vi "S8300E_Chk_TEMPERATURE_WIH.vi"() -> ()   [LabVIEW 2011]
uses:
  Instance          16 28Saved   KT300WR2_TP125B_PCBA .vi
  Instance          20 28Saved   KT300WR2_TP125B_PCBA .vi
panel:
  out "history_log":string
  out "VISA resource name out":refnum<visa-resource-name>
  out "SEARCHING Test Item":string[](array[string])
  out "SFCS_Network Ok?":bool=TRUE
  out "log_measured Voltage":string
  out "begin time":u32
  out "All Pass?":bool=TRUE
  out "Result(測試總結果)":bool
  out "Total TP":i32
  out "record(s)":T1(array[cluster])
  out "狀況":string
  out "Test Result (測試結果)":T2(array[cluster])
  # "S8300E 溫度Test Points Check"
  # "2015-6-1"
  # "Error Code\nCPU1\nCPU2\nPCH\nDDR3-1T\nDDR3-2T\nMB"
types:
  T1 = cluster{"TestPoint_Name":string, "Lower Limit Voltage":dbl, "High Limit Voltage":dbl, cluster{"Relay3 Name":string, "Relay3H/L":bool}[], "Measure Ai name":string}[]
  T2 = cluster{"Test Item":string, "SPEC MIN C":dbl, "SPEC MAX C":dbl, "Measured C":dbl, bool}[]
  T3 = enum16{"open", "replace", "create", "open or create", "replace or create", "replace or create with confirmation"}
  T4 = cluster{"Test Item":string, "SPEC MIN V":dbl, "SPEC MAX V":dbl, "Measured V":dbl, bool}[]
  T5 = cluster{"Test Item":string, "SPEC MIN C":dbl, "SPEC MAX C":dbl, "Measured C":dbl, bool}
  T6 = cluster{"TestPoint_Name":string, "Lower Limit Voltage":dbl, "High Limit Voltage":dbl, cluster{"Relay3 Name":string, "Relay3H/L":bool}[], "Measure Ai name":string}
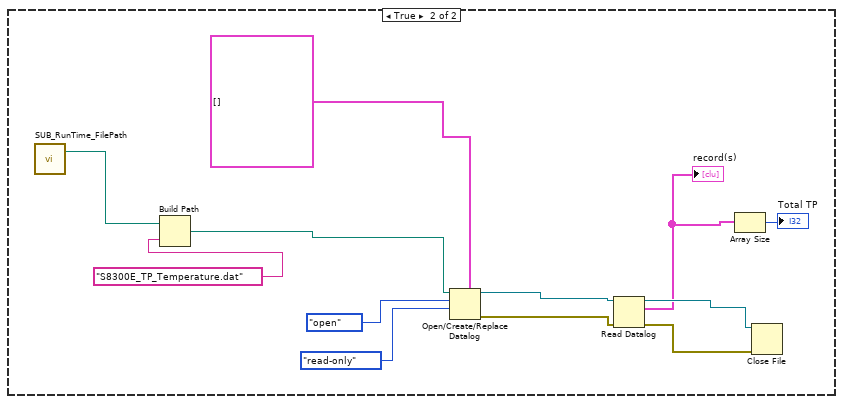
[diagram p2: hidden frame]
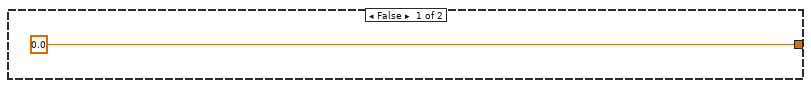
[diagram p6: hidden frame]
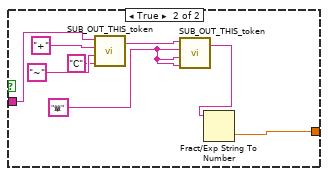
[diagram p7: hidden frame]
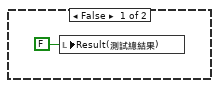
[diagram p9: hidden frame]
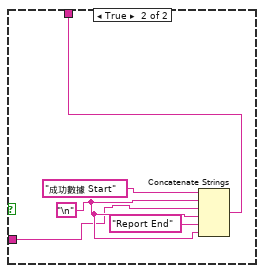
[diagram p10: hidden frame]
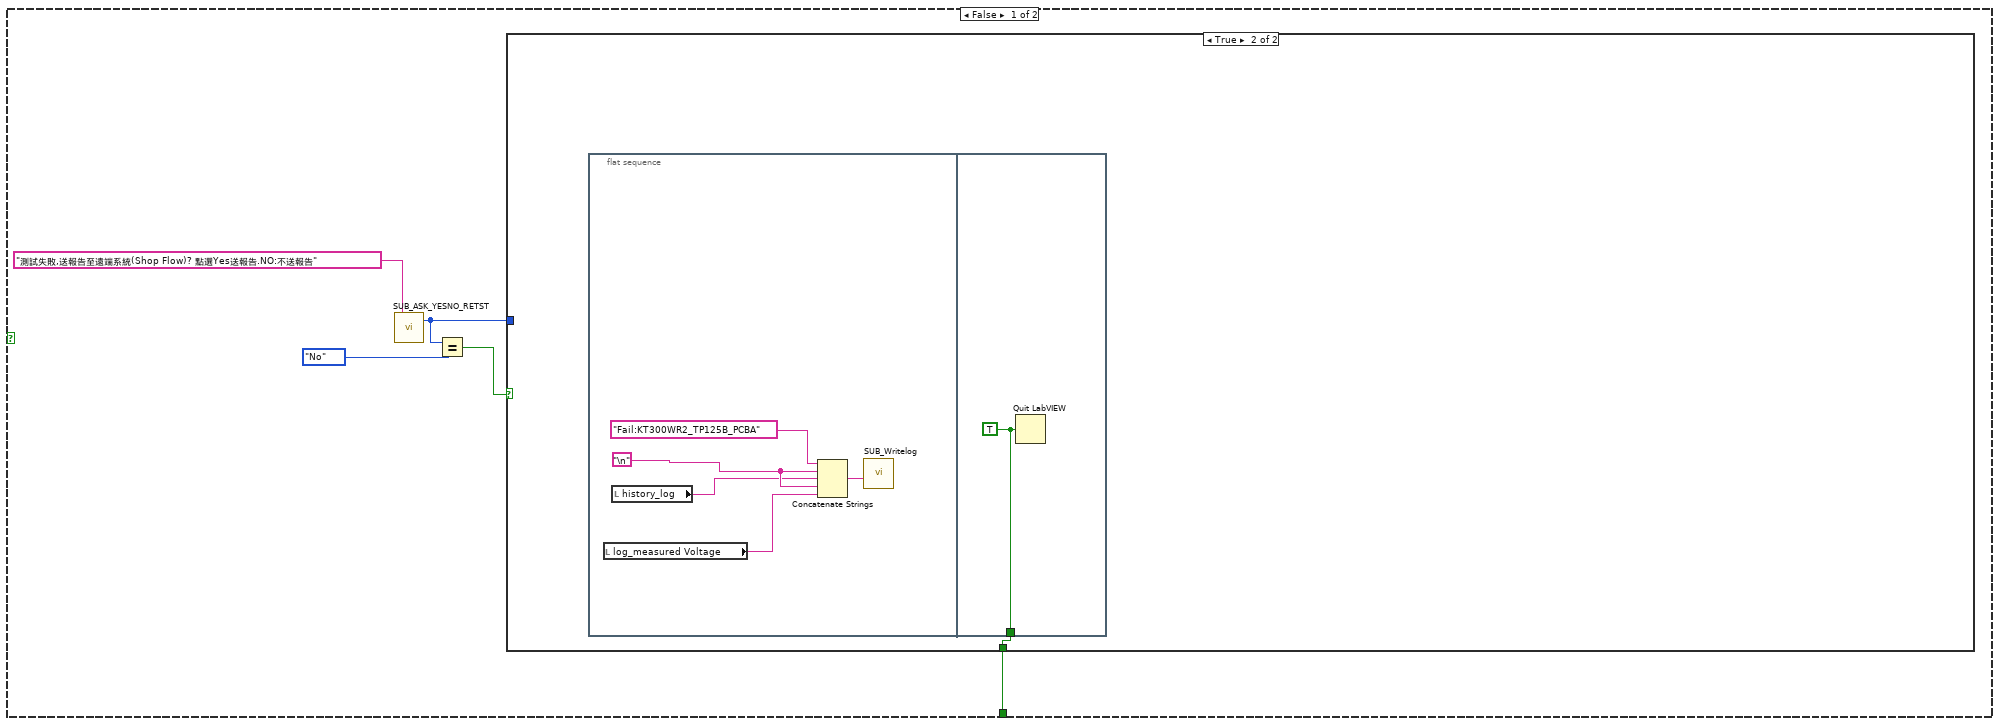
[diagram p11: hidden frame]
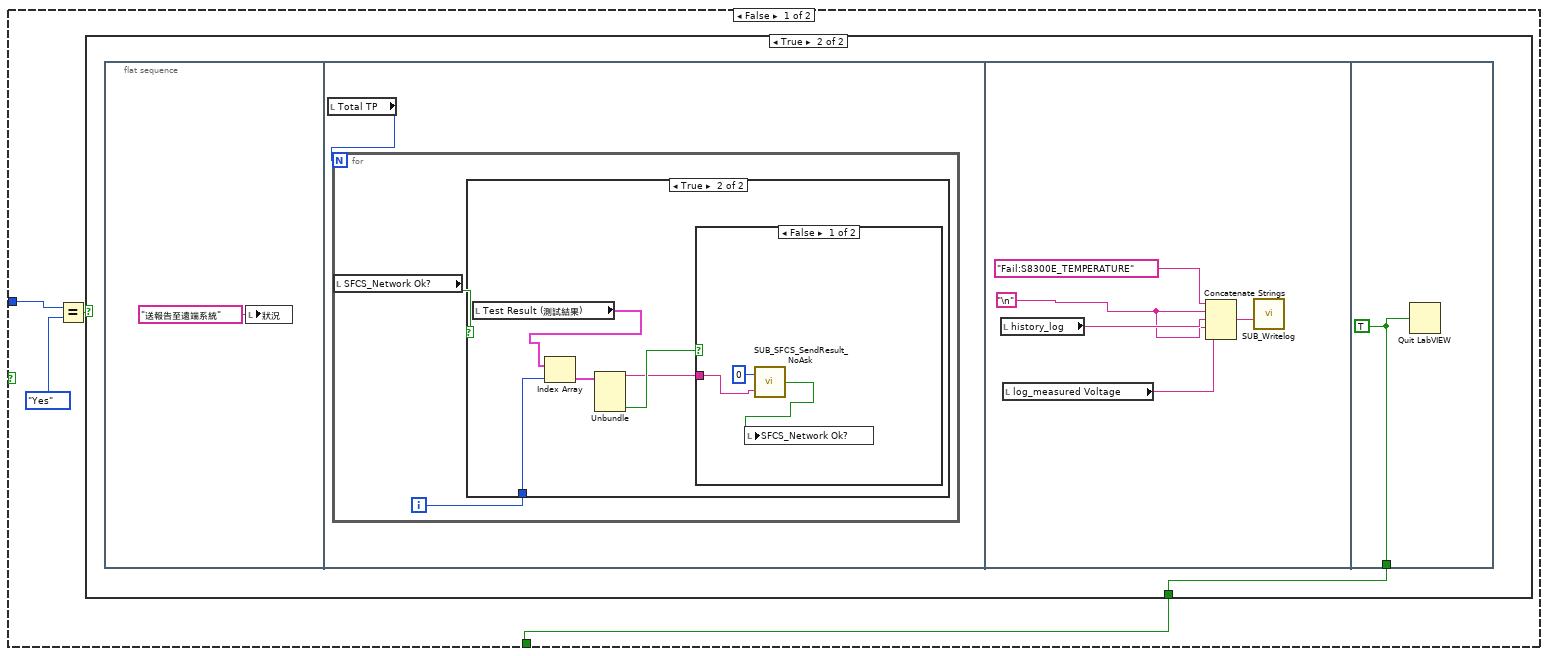
[diagram p12: hidden frame]
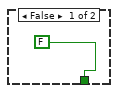
[diagram p13: hidden frame]
diagram:
  n1 = while {
    shift-right: [w4] -> _
    shift-left: "" -> [w3]
    stop <- w6 stop-if-true
    n2 = flat-sequence {
      tunnel: [w48] -> w5
      tunnel: w5 -> [w75]
      tunnel: [w167] -> w2
      tunnel: [w182] -> w6
      frame #0 {
        n3 = Tick Count (ms)() -> (millisecond timer value=→"begin time":u32)
      }
      frame #1 {
        n4 = property on="Result(測試總結果)" class="Bool (strict)"("Visible"=FALSE) -> ()  [unwired: 2 in, 2 out]
        n5 = property on="狀況" class="Str"("Blinking"=TRUE) -> ()  [unwired: 2 in, 2 out]
        "SFCS_Network Ok?" <- TRUE
        "狀況" <- ""
        "Result(測試總結果)" <- FALSE ("Result(測試總結果)")
        "All Pass?" <- TRUE
      }
      frame #2 {
        n6 = call "SUB_SearchFile_inFolder.vi"("Search Filename in Folder"="S8300E_TP_Temperature.dat" ("name or relative path")) -> ("File Existing True/Flase"=w14:bool)  [unwired: 1 in]
        n7 = case shown="False" w14 {
          frame False {
            n8 = flat-sequence {
              frame #0 {
                n9 = call "Display Message to User"() -> ()  [unwired: 10 in, 2 out]
              }
              frame #1 {
                n10 = call "SUB_Writelog.vi"("Pass/Fail"="Fail:S8300E_Chk_TEMPERATURE") -> ()  [unwired: 2 in]
              }
              frame #2 {
                n11 = Quit LabVIEW(quit? (T)=TRUE) -> ()
              }
            }
          }
          frame True {
            n12 = call "SUB_RunTime_FilePath.vi"() -> ("stripped path"=w19:path)  [unwired: 3 in]
            n13 = Build Path(base path=w19, name or relative path="S8300E_TP_Temperature.dat") -> (appended path=w26:path)
            n14 = Open/Create/Replace Datalog(5:T1 [] ("DatalogType"), 9:enum16{"read/write", "read-only", "write-only"}."read-only" ("access (0:read/write)"), 10:T3."open" ("operation (0:open)"), 11:w26) -> (0:w23:errorcluster, 3:w22:refnum<k1>)  [unwired: 2 in, 1 out]
            n15 = Read Datalog(4:w23, 7:w22) -> (0:w25:errorcluster, 2:w21:T1, 3:w24:refnum<k1>)  [unwired: 1 in]
            "record(s)" <- w21
            n16 = Array Size(array=w21) -> (size(s)=→"Total TP":i32)
            n17 = Close File(refnum=w24, error in=w25) -> ()  [unwired: 2 out]
          }
        }
      }
      frame #3 {
        # "這邊只是示範,如何從Records 找出欲測測點的\n資料"
        n18 = Build Array("CPU1", "CPU2", "PCH " ("TestPoint_Name"), "DDR3-1T" ("TestPoint_Name"), "DDR3-2T" ("TestPoint_Name"), "MB" ("TestPoint_Name")) -> (w36:string[])
        "SEARCHING Test Item" <- w36
        n19 = Array Size(array=w36) -> (size(s)=w35:i32)
        n20 = local write "Total TP"(w35) -> ()
      }
      frame #4 {
        n21 = local read "Total TP"() -> (w40:i32)
        n22 = for {
          N: w40 -> [_]
          shift-right: [w43] -> w38
          shift-left: T4 [] -> [w41]
          n23 = call "SUB_TP_Output.vi"("Measured C"=-1.0 ("Measured V"), "SPEC MAX C"=0.0 ("SPEC MAX V"), "SPEC MIN C"=0.0 ("SPEC MIN V"), "Test Item"="") -> ("result"=w42:T5)  [unwired: 2 out]
          n24 = Build Array (concatenate)(w41, w42) -> (w43:T2)
        }
        "Test Result (測試結果)" <- w38
      }
      frame #5 {
        n25 = local read "Total TP"() -> (w50:i32)
        n26 = for {
          N: w50 -> [_]
          shift-right: [w52] -> w48
          shift-left: T1 [] -> [w51]
          i -> [w57]
          n27 = local read "SEARCHING Test Item"() -> (w58:string[])
          n28 = Index Array(array=w58, index=w57) -> (element=w55:string)
          n29 = call <vilib>:"Trim Whitespace.vi"("string"=w55) -> ("trimmed string"=w56:string)  [unwired: 1 in]
          n30 = To Upper Case(1:w56) -> (0:w54:string)
          n31 = while {
            tunnel: w54 -> [w64]
            tunnel: [w62] -> w53
            i -> [w59]
            stop <- w70 stop-if-true
            n32 = local read "record(s)"() -> (w68:T1)
            n33 = Array Size(array=w68) -> (size(s)=w60:i32)
            n34 = Index Array(array=w68, index=w59) -> (element=w61:T6)
            n35 = Unbundle By Name(w61) -> ("TestPoint_Name"=w67:string)
            n36 = call <vilib>:"Trim Whitespace.vi"("string"=w67) -> ("trimmed string"=w66:string)  [unwired: 1 in]
            n37 = To Upper Case(1:w66) -> (0:w65:string)
            n38 = Greater Or Equal?(x=w59, y=w60) -> (x >= y?=w69:bool)
            n39 = Equal?(x=w65, y=w64) -> (x = y?=w63:bool)
            n40 = case shown="True" w63 {
              tunnel: [_ w71] -> w62
              tunnel: w61 -> [_ w71]
              frame False {
              }
              frame True {
              }
            }
            n41 = Or(x=w63, y=w69) -> (x .or. y?=w70:bool)
          }
          n42 = Build Array (concatenate)(w51, w53) -> (w52:T1)
        }
        n43 = local write "record(s)"(w48) -> ()
      }
      frame #6 {
        n44 = local read "Total TP"() -> (w73:i32)
        n45 = Array Size(array=w75) -> (size(s)=w72:i32)
        n46 = Not Equal?(x=w72, y=w73) -> (x != y?=w74:bool)
        n47 = case shown="True" w74 {
          tunnel: w73 -> [_ w77]
          tunnel: w72 -> [_ w76]
          frame False {
          }
          frame True {
            n48 = flat-sequence {
              tunnel: w77 -> [w89]
              tunnel: w76 -> [w83]
              frame #0 {
                n49 = Number To Decimal String(number=w89) -> (decimal integer string=w87:string)  [unwired: 1 in]
                n50 = Number To Decimal String(number=w83) -> (decimal integer string=w82:string)  [unwired: 1 in]
                n51 = Concatenate Strings("失敗!", "需找", w87, "筆", "\r", "但實際上找找到", w82, "筆", "\r") -> (w79:string)
                n52 = call "Display Message to User3"("Message"=w79) -> ()  [unwired: 9 in, 2 out]
              }
              frame #1 {
                n53 = call "SUB_Writelog.vi"("Pass/Fail"="Fail:S8300E_Chk_TEMPERATURE") -> ()  [unwired: 2 in]
              }
              frame #2 {
                n54 = Quit LabVIEW(quit? (T)=TRUE) -> ()
              }
            }
          }
        }
      }
      frame #7 {
        n55 = call "SUB_COM1_CLOSE.vi"("VISA resource name"=refnum<visa-resource-name> "COM9") -> ()  [unwired: 3 in]
      }
      frame #8 {
        n56 = case shown="True" TRUE {
          frame False {
          }
          frame True {
            n57 = call "SUB_COM9_INIT.vi"("baud rate"=u32 115200) -> ("VISA resource name out"=w97:refnum<visa-resource-name>)  [unwired: 1 in, 1 out]
            "VISA resource name out" <- w97
            n58 = call "SUB_COM1Wrt.vi"("VISA resource name"=w97, "write buffer"="\r") -> ("duplicate VISA resource name"=w94:refnum<visa-resource-name>)  [unwired: 1 in, 1 out]
            n59 = call "SUB_ContinueCom1Read.vi"("Numeric"=1200, "duplicate VISA resource name 2"=w94) -> ()  [unwired: 1 in, 3 out]
          }
        }
      }
      frame #9 {
        n60 = local read "Total TP"() -> (w101:i32)
        n61 = for {
          N: w101 -> [_]
          shift-right: [w107] -> w99
          shift-left: "" -> [w106]
          i -> [w108]
          n62 = flat-sequence {
            tunnel: w108 -> [w116]
            tunnel: [w111] -> w105
            tunnel: [w109] -> w104
            tunnel: [w110] -> w103
            tunnel: [w112] -> w102
            tunnel: w108 -> [w134]
            tunnel: w105 -> [w121]
            tunnel: w104 -> [w132]
            tunnel: w103 -> [w131]
            tunnel: [w126] -> w107
            tunnel: w106 -> [w125]
            tunnel: w102 -> [w123]
            frame #0 {
              n63 = local read "record(s)"() -> (w117:T1)
              n64 = Index Array(array=w117, index=w116) -> (element=w113:T6)
              n65 = Unbundle By Name(w113) -> ("TestPoint_Name"=w111:string, "Lower Limit Voltage"=w109:dbl, "High Limit Voltage"=w110:dbl, "Measure Ai name"=w112:string)
              n66 = Concatenate Strings(w111, "  測點測試中..." ("string")) -> (w115:string)
              n67 = local write "狀況"(w115) -> ()
            }
            frame #1 {
              n68 = case shown="True" TRUE {
                tunnel: [0.0 ("AVG_Vol") w146] -> w124
                tunnel: w123 -> [_ w147]
                frame False {
                }
                frame True {
                  n69 = local read "VISA resource name out"() -> (w143:refnum<visa-resource-name>)
                  n70 = Concatenate Strings(w147, "\r") -> (w142:string)
                  n71 = Tick Count (ms)() -> (millisecond timer value=w138:u32)
                  n72 = call "SUB_WR_COM1_CbyCFindString_timeout.vi"("Begin time"=w138, "Find this String"=";", "Timeout Seccond"=3.0, "cmd string"=w142, "duplicate VISA resource name 2"=w143) -> ("Output String"=w139:string)  [unwired: 3 out]
                  n73 = call "SUB_FindSpecificString.vi"("Find this String"="PASSED=", "String data"=w139) -> ("before \"; \" string"=w145:string, "Found"=w144:bool)  [unwired: 2 in]
                  n74 = case shown="False" w144 {
                    tunnel: w145 -> [_ w156]
                    tunnel: [999.0 w157] -> w146
                    frame False {
                    }
                    frame True {
                      w151 = "簞"
                      n75 = call "SUB_OUT_THIS_token.vi"("Remove token symbl1 3"="C", "Remove token symbl1 2"="~", "Remove token symbl1"="+", "input string"=w156) -> ("result string"=w152:string)  [unwired: 1 in]
                      n76 = call "SUB_OUT_THIS_token.vi"("Remove token symbl1 3"=w151, "Remove token symbl1 2"=w151, "Remove token symbl1"=w151, "input string"=w152) -> ("result string"=w150:string)  [unwired: 1 in]
                      n77 = Fract/Exp String To Number(string=w150) -> (number=w157:dbl)  [unwired: 3 in, 1 out]
                    }
                  }
                }
              }
              n78 = local read "Test Result (測試結果)"() -> (w135:T2)
              n79 = call "SUB_TP_Output.vi"("Measured C"=w124, "SPEC MAX C"=w131, "SPEC MIN C"=w132, "Test Item"=w121) -> ("result"=w130:T5)  [unwired: 2 out]
              n80 = Number To Fractional String(number=w124, precision (6)=i16 2) -> (F-format string=w128:string)  [unwired: 2 in]
              n81 = Replace Array Subset(array=w135, new element=w130, index=w134) -> (w133:T2)
              n82 = local write "Test Result (測試結果)"(w133) -> ()
              n83 = Concatenate Strings(w121, " Temp=" ("string"), w128, ";", "\n") -> (w127:string)
              n84 = Concatenate Strings(w125, w127) -> (w126:string)
            }
          }
        }
        "log_measured Voltage" <- w99
      }
      frame #10 {
        n85 = local read "Total TP"() -> (w158:i32)
        n86 = for {
          N: w158 -> [_]
          i -> [w161]
          n87 = local read "Test Result (測試結果)"() -> (w162:T2)
          n88 = Index Array(array=w162, index=w161) -> (element=w160:T5)
          n89 = Unbundle(w160) -> (w159:bool)  [unwired: 4 out]
          n90 = case shown="False" w159 {
            frame False {
              n91 = local write "All Pass?"(FALSE ("All Pass?")) -> ()
            }
            frame True {
            }
          }
        }
      }
      frame #11 {
        n92 = local read "All Pass?"() -> (w164:bool)
        n93 = case shown="True" w164 {
          frame False {
            n94 = local write "Result(測試總結果)"(FALSE ("Result(測試總結果)")) -> ()
          }
          frame True {
            n95 = local write "Result(測試總結果)"(TRUE ("Result(測試總結果)")) -> ()
          }
        }
      }
      frame #12 {
        n96 = local read "log_measured Voltage"() -> (w168:string)
        n97 = local read "All Pass?"() -> (w169:bool)
        n98 = case shown="False" w169 {
          tunnel: w168 -> [w173 w176]
          tunnel: [w170 w175] -> w167
          frame False {
            w171 = "\n"
            n99 = Concatenate Strings("失敗數據 Start" ("string"), w171, w173, w171, "Report End" ("string"), w171) -> (w170:string)
          }
          frame True {
            w177 = "\n"
            n100 = Concatenate Strings("成功數據 Start" ("string"), w177, w176, w177, "Report End" ("string"), w177) -> (w175:string)
          }
        }
      }
      frame #13 {
        n101 = local write "SFCS_Network Ok?"(TRUE ("SFCS_Network Ok?")) -> ()
        n102 = property on="Result(測試總結果)" class="Bool (strict)"("Visible"=TRUE) -> ()  [unwired: 2 in, 2 out]
      }
      frame #14 {
        n103 = local read "All Pass?"() -> (w183:bool)
        n104 = case shown="True" w183 {
          tunnel: [w185 _] -> w182
          frame False {
            n105 = call "SUB_ASK_YESNO_RETST.vi"("Question:"="測試失敗,送報告至遠端系統(Shop Flow)? 點選Yes送報告.NO:不送報告") -> ("yes/no"=w184:enum32{"No Selection", "Yes", "No", "None"})  [unwired: 2 in]
            n106 = Equal?(x=w184, y=enum32{"No Selection", "Yes", "No", "None"}."No") -> (x = y?=w186:bool)
            n107 = case shown="True" w186 {
              tunnel: [w192 w213] -> w185
              tunnel: w184 -> [w190 _]
              frame False {
                n108 = Equal?(x=w190, y=enum32{"No Selection", "Yes", "No", "None"}."Yes") -> (x = y?=w191:bool)
                n109 = case shown="True" w191 {
                  tunnel: [FALSE w194] -> w192
                  frame False {
                  }
                  frame True {
                    n110 = flat-sequence {
                      tunnel: [w212] -> w194
                      frame #0 {
                        n111 = local write "狀況"("送報告至遠端系統" ("狀況")) -> ()
                      }
                      frame #1 {
                        n112 = local read "Total TP"() -> (w196:i32)
                        n113 = for {
                          N: w196 -> [_]
                          i -> [w198]
                          n114 = local read "SFCS_Network Ok?"() -> (w197:bool)
                          n115 = case shown="True" w197 {
                            tunnel: w198 -> [_ w202]
                            frame False {
                            }
                            frame True {
                              n116 = local read "Test Result (測試結果)"() -> (w203:T2)
                              n117 = Index Array(array=w203, index=w202) -> (element=w201:T5)
                              n118 = Unbundle(w201) -> ("Test Item"=w199:string, w200:bool)  [unwired: 3 out]
                              n119 = case shown="False" w200 {
                                tunnel: w199 -> [w205 _]
                                frame False {
                                n120 = call "SUB_SFCS_SendResult_NoAsk.vi"("ErrorCode"=w205, "PASS_Fail (1/0)"=i8 0) -> ("Sent OK ?"=w204:bool)
                                n121 = local write "SFCS_Network Ok?"(w204) -> ()
                                }
                                frame True {
                                }
                              }
                            }
                          }
                        }
                      }
                      frame #2 {
                        w208 = "\n"
                        n122 = local read "history_log"() -> (w209:string)
                        n123 = local read "log_measured Voltage"() -> (w207:string)
                        n124 = Concatenate Strings("Fail:S8300E_TEMPERATURE", w208, w209, w208, w207) -> (w211:string)
                        n125 = call "SUB_Writelog.vi"("Pass/Fail"=w211) -> ()  [unwired: 2 in]
                      }
                      frame #3 {
                        w212 = TRUE ("quit? (T)")
                        n126 = Quit LabVIEW(quit? (T)=w212) -> ()
                      }
                    }
                  }
                }
              }
              frame True {
                n127 = flat-sequence {
                  tunnel: [w219] -> w213
                  frame #0 {
                    w216 = "\n"
                    n128 = local read "log_measured Voltage"() -> (w214:string)
                    n129 = local read "history_log"() -> (w215:string)
                    n130 = Concatenate Strings("Fail:KT300WR2_TP125B_PCBA", w216, w215, w216, w214) -> (w218:string)
                    n131 = call "SUB_Writelog.vi"("Pass/Fail"=w218) -> ()  [unwired: 2 in]
                  }
                  frame #1 {
                    w219 = TRUE ("quit? (T)")
                    n132 = Quit LabVIEW(quit? (T)=w219) -> ()
                  }
                }
              }
            }
          }
          frame True {
            n133 = flat-sequence {
              frame #0 {
                n134 = call "SUB_COM1_CLOSE.vi"("VISA resource name"=refnum<visa-resource-name> "COM9") -> ()  [unwired: 3 in]
              }
              frame #1 {
                w223 = "***Not Good ***" ("replace string (\"\")")
                w228 = "\n"
                n135 = local read "history_log"() -> (w229:string)
                n136 = local read "begin time"() -> (w233:u32)
                n137 = Tick Count (ms)() -> (millisecond timer value=w232:u32)
                n138 = call "SUB_CAL_TESTTIME.vi"("Test Item name"="S8300E_Chk_TEMPERATURE", "Stop tick time"=w232, "Start tick time"=w233) -> ("Test Time output"=w227:string)  [unwired: 2 in]
                n139 = Concatenate Strings("Pass:S8300E_Chk_TEMPERATURE", w228, w229, w228, w227) -> (w222:string)
                n140 = call "SUB_SEARCH_REPLACE_STR.vi"("replace string (\"\")"=w223, "search string"="FAILED", "input string"=w222) -> ("result string"=w225:string)  [unwired: 2 in]
                n141 = call "SUB_SEARCH_REPLACE_STR.vi"("replace string (\"\")"=w223, "search string"="FAIL", "input string"=w225) -> ("result string"=w221:string)  [unwired: 2 in]
                n142 = call "SUB_Writelog.vi"("Pass/Fail"=w221) -> ()  [unwired: 2 in]
              }
              frame #2 {
                n143 = Request Deallocation(TRUE ("flag")) -> ()
              }
              frame #3 {
                n144 = Quit LabVIEW(quit? (T)=TRUE) -> ()
              }
            }
          }
        }
      }
    }
    n145 = Concatenate Strings(w3, w2) -> (w4:string)
    "history_log" <- w4
  }
